vi "LoadNISTWfrmPlugin.vi"(8 "ErrorArray In":errorcluster[](array[cluster]), 10 "clBusData In":T1, 11 "NISTBus In":refnum<class "NISTBus.lvclass">) -> (0 "ErrorArray Out":errorcluster[](array[cluster]), 2 "clBusData Out":T1, 3 "NISTBus Out":refnum<class "NISTBus.lvclass">)   [LabVIEW 2014, in "Bus.lvlib" / "NISTBus.lvclass"]
uses:
  NISTBus.lvclass
  TypeDefs/clBusData.ctl
  FGenPlugins/MyPluginBaseClass/TypeDef/PluginParams.ctl
  <userlib>/NIST/NISTErrorLib/NISTErrorLib.lvlib
  WfrmGenerator/WfrmModule/WfrmModule.lvlib
  FGenPlugins/MyPluginBaseClass/NISTFGenPluginsBase.lvclass
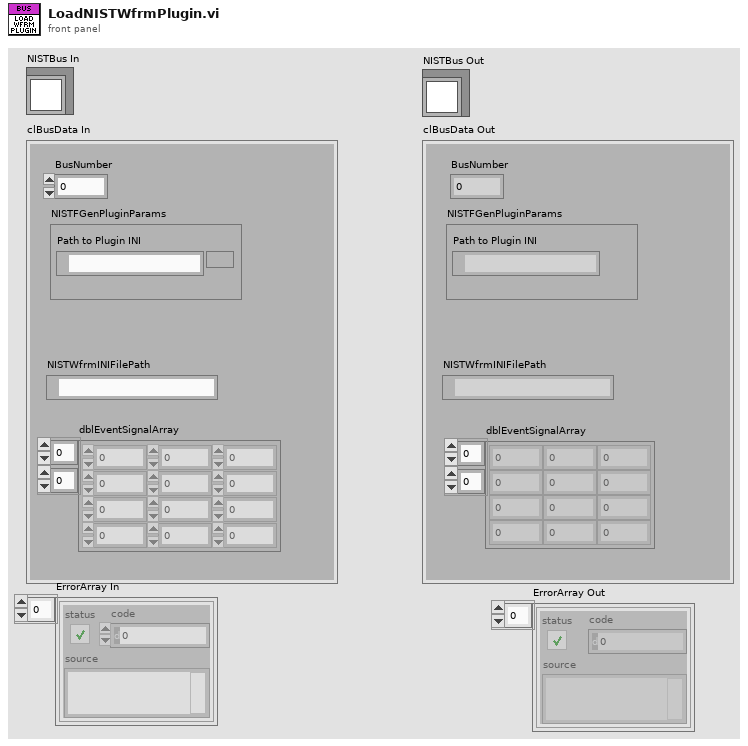
[diagram p1: front panel]
types:
  T1 = typedef "Bus.lvlib/NISTBus.lvclass/clBusData.ctl" = cluster{"BusNumber":u8, "NISTWfrmINIFilePath":path, "dblEventSignalArray":dbl[][], "NISTFGenPluginParams":T2}
  T2 = typedef "FGenPlugins.lvlib/NISTFGenPluginsBase.lvclass/PluginParams.ctl" = cluster{"Path to Plugin INI":path}
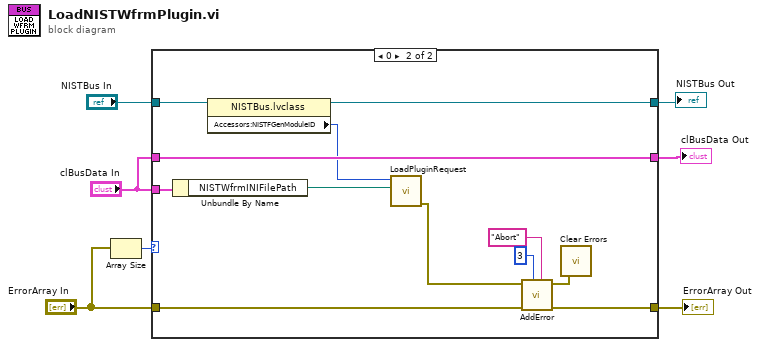
[diagram p0: block diagram]
diagram:
  n1 = Array Size(array="ErrorArray In") -> (size(s)=w7:i32)
  n2 = case shown="0" w7 {
    tunnel: [w10 w16] -> w6
    tunnel: "ErrorArray In" -> [w10 w17]
    tunnel: "clBusData In" -> [_ w22]
    tunnel: "NISTBus In" -> [w9 w21]
    tunnel: [w8 w15] -> w3
    tunnel: "clBusData In" -> [w8 w15]
    tunnel: [w9 w14] -> w1
    frame 1, Default {
    }
    frame 0 {
      n3 = Unbundle By Name(w22) -> ("NISTWfrmINIFilePath"=w12:path)
      n4 = property class="NISTBus.lvclass"(reference=w21) -> (reference out=w14:refnum<class "NISTBus.lvclass">, "Accessors:NISTFGenModuleID"=w11:i32)  [unwired: 1 in, 1 out]
      n5 = call "LoadPluginRequest.vi"("PathToPlugin"=w12, "ModuleID"=w11) -> ("error out"=w13:errorcluster)  [unwired: 9 in]
      n6 = call <userlib>:"AddError.vi"("Severity"="Abort" ("String"), "Priority"=u8 3, "ErrorArray"=w17, "error in (no error)"=w13) -> ("ErrorArray"=w16:errorcluster[], "error out"=w18:errorcluster)  [unwired: 6 in]
      n7 = call <vilib>:"Clear Errors.vi"("error in (no error)"=w18) -> ()  [unwired: 5 in, 2 out]
    }
  }
  "clBusData Out" <- w3
  "NISTBus Out" <- w1
  "ErrorArray Out" <- w6
